vi "Test Remove Empty String.vi"(8 "error in (no error)":errorcluster, 11 "LUnit Test Suite Tests in":refnum<class "LUnit Test Suite Tests.lvclass">) -> (0 "error out":errorcluster, 3 "LUnit Test Suite Tests out":refnum<class "LUnit Test Suite Tests.lvclass">)   [LabVIEW 2020, in "LUnit Test Suite Tests.lvclass"]
uses:
  LUnit Test Suite Tests.lvclass
  LUnit Test Suite Tests.lvclass/LUnit Test Suite Tests.ctl
  source/LUnit Test Suite.lvclass
  Test Doubles/Test Case Test Double/Test Case Test Double.lvclass
  <vilib>/Astemes/LUnit/Test Case.lvclass
panel:
  out "List of Runnables":string[](array[string])
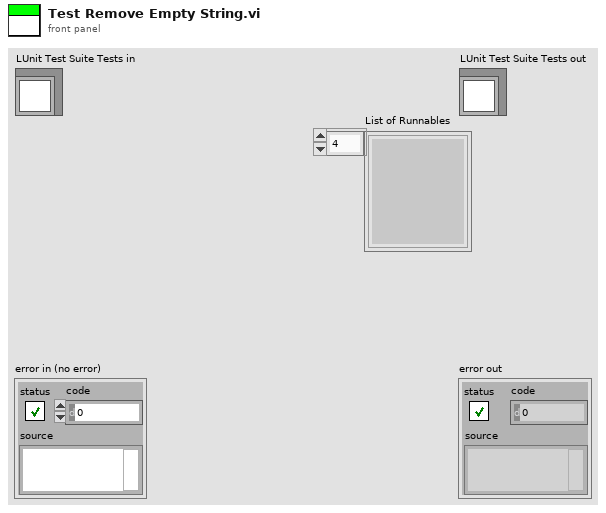
[diagram p1: front panel]
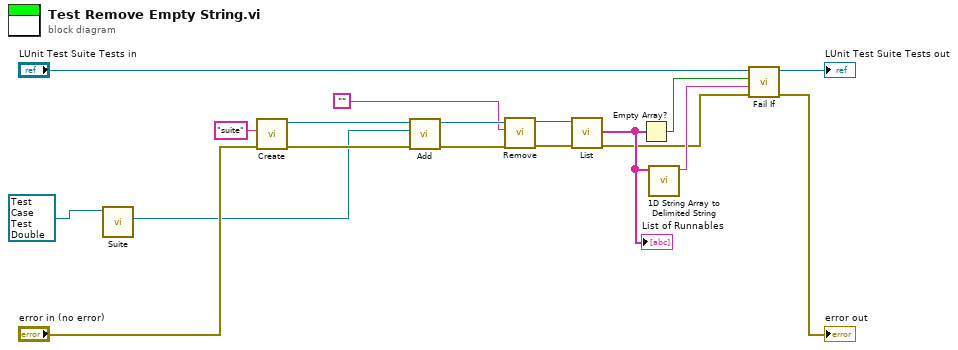
[diagram p0: block diagram]
diagram:
  n1 = call-dynamic "Suite.vi"("LUnit Test Case In"=refnum<class "Test Case Test Double.lvclass"> refnum ("Test Case Test Double.lvclass")) -> ("LUnit Test Suite Out"=w2:refnum<class "LUnit Test Suite.lvclass">)  [unwired: 8 in, 2 out]
  n2 = call "Create.vi"("error in (no error)"="error in (no error)", "Suite Name"="suite") -> ("error out"=w16:errorcluster, "LUnit Test Suite Out"=w17:refnum<class "LUnit Test Suite.lvclass">)  [unwired: 8 in]
  n3 = call "Add.vi"("error in (no error)"=w16, "Runnable"=w2, "LUnit Test Suite In"=w17) -> ("error out"=w14:errorcluster, "LUnit Test Suite Out"=w15:refnum<class "LUnit Test Suite.lvclass">)  [unwired: 7 in]
  n4 = call "Remove.vi"("error in (no error)"=w14, "Test to Remove"="", "LUnit Test Suite In"=w15) -> ("error out"=w12:errorcluster, "LUnit Test Suite Out"=w13:refnum<class "LUnit Test Suite.lvclass">)  [unwired: 7 in]
  n5 = call "List.vi"("error in (no error)"=w12, "LUnit Test Suite In"=w13) -> ("error out"=w5:errorcluster, "List of Runnables"=w7:string[])  [unwired: 8 in]
  "List of Runnables" <- w7
  n6 = Empty Array?(array=w7) -> (empty?=w8:bool)
  n7 = call <vilib>:"1D String Array to Delimited String.vi"("string array"=w7) -> ("delimited string"=w6:string)  [unwired: 10 in]
  n8 = call <vilib>:"Fail If.vi"("error in (no error)"=w5, "Message"=w6, "Fail?"=w8, "LUnit Test Case In"="LUnit Test Suite Tests in") -> ("error out"=→"error out":errorcluster, "LUnit Test Case Out"=→"LUnit Test Suite Tests out":refnum<class "LUnit Test Suite Tests.lvclass">)  [unwired: 6 in]
